vi "DAQ_Configure.vi"(6 "Dwell time (µs)":dbl, 7 "Scan XY (T) / i(t) (F)":bool, 8 "error in":errorcluster caption="entrée d'erreur", 9 "Position XY (for i(t))":dbl[](array[numeric]), 10 "Scanning positions":dbl[][](array[numeric]), 11 "Scanning cluster":T2={"Nx"=4, "Ny"=4, "# Repetition"=1, "FOV_X (µm)"=100.0, "FOV_Y (µm)"=100.0, "Calib_X"=0.1, "Calib_Y"=0.1, "Center X (µm)"=50.0, "Center_Y (µm)"=50.0, "Bi-directionnal?"=FALSE} {"# Repetition" min=1 step=1; "Ny" min=1 step=1; "Nx" min=1 step=1}) -> (0 "error out":errorcluster caption="sortie d'erreur", 3 "Task cluster":T1)   [LabVIEW 2026]
uses:
  <vilib>/DAQmx/write.llb/DAQmx Write (Analog 1D DBL NChan 1Samp).vi
  <vilib>/DAQmx/write.llb/DAQmx Write (Analog 2D DBL NChan NSamp).vi
  <vilib>/DAQmx/create/channels.llb/DAQmx Create Channel (CO-Pulse Generation-Frequency).vi
  <vilib>/DAQmx/configure/timing.llb/DAQmx Timing (Implicit).vi
  <vilib>/DAQmx/create/channels.llb/DAQmx Create Channel (AO-Voltage-Basic).vi
  <vilib>/DAQmx/miscellaneous.llb/DAQmx Fill In Error Info.vi
  <vilib>/DAQmx/configure/timing.llb/DAQmx Timing (Sample Clock).vi
  <vilib>/DAQmx/create/channels.llb/DAQmx Create Channel (AI-Voltage-Basic).vi
  <vilib>/DAQmx/configure/trigger.llb/DAQmx Start Trigger (Digital Edge).vi
  <vilib>/DAQmx/create/channels.llb/DAQmx Create Channel (CI-Pulse Width).vi
  <resource>/objmgr/daqmx.rc
panel:
  out "Pixel_Freq":dbl
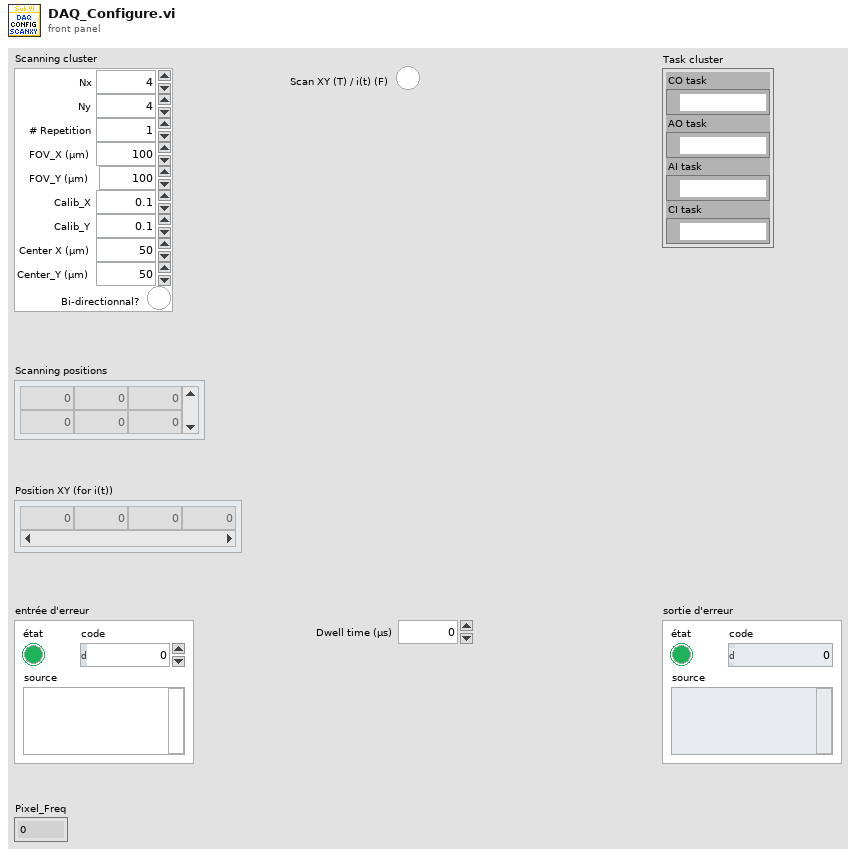
[diagram p1: front panel]
types:
  T1 = cluster{"CO task":refnum<k21>, "AO task":refnum<k21>, "AI task":refnum<k21>, "CI task":refnum<k21>}
  T2 = cluster{"Nx":u16, "Ny":u16, "# Repetition":u16, "FOV_X (µm)":dbl, "FOV_Y (µm)":dbl, "Calib_X":dbl, "Calib_Y":dbl, "Center X (µm)":dbl, "Center_Y (µm)":dbl, "Bi-directionnal?":bool}
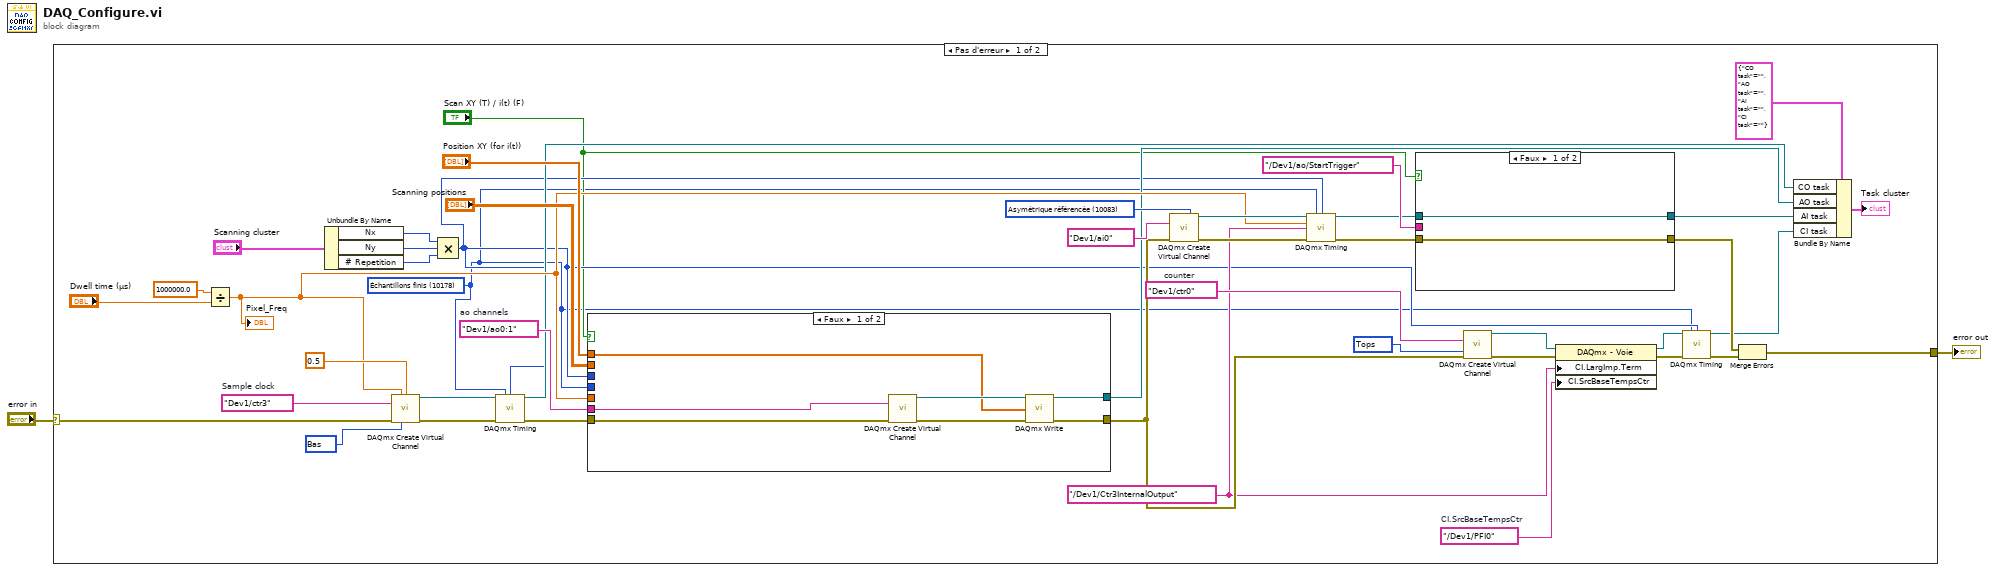
[diagram p0: block diagram]
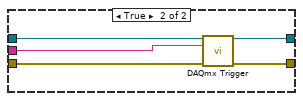
[diagram p2: hidden frame]
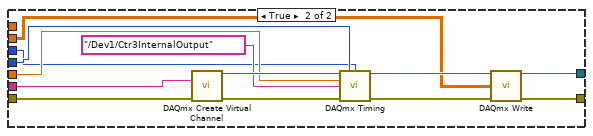
[diagram p3: hidden frame]
diagram:
  n1 = case shown="Pas d'erreur" "error in" {
    selector: "error in" -> [w45 w75]
    tunnel: [w19 w75] -> w1
    frame No Error {
      w15 = tag "/Dev1/PFI0"  # CI.SrcBaseTempsCtr
      w23 = 10304 items=["Secondes"=10364, "Tops"=10304, "D'une échelle personnalisée"=10065] ("units")
      w24 = tag "Dev1/ctr0"  # counter
      w18 = tag "/Dev1/Ctr3InternalOutput" ("source")
      w30 = 10083 items=["Par défaut"=-1, "Asymétrique référencée"=10083, "Asymétrique non référencée"=10078, "Différentielle"=10106, "Pseudodifférentielle"=12529] ("input terminal configuration")
      w37 = tag "Dev1/ao0:1"  # ao channels
      w3 = 10178 items=["Échantillons finis"=10178, "Échantillons continus"=10123, "Point par point avec cadencement matériel"=12522] ("sample mode")
      w40 = 10214 items=["Haut"=10192, "Bas"=10214] ("idle state")
      w42 = tag "Dev1/ctr3"  # Sample clock
      n2 = Divide(x=1000000.0, y="Dwell time (µs)") -> (x/y=w27:dbl)
      "Pixel_Freq" <- w27
      n3 = Unbundle By Name("Scanning cluster") -> ("Nx"=w34:u16, "Ny"=w33:u16, "# Repetition"=w32:u16)
      n4 = call-poly <vilib>:"DAQmx Create Virtual Channel.vi"("frequency"=w27, "duty cycle"=0.5 ("Duty cycle"), "counter"=w42, "error in"=w45, "idle state"=w40) -> ("task out"=w44:refnum<k21>, "error out"=w43:errorcluster)  [unwired: 9 in]
      n5 = Compound Arithmetic op=MULTIPLY(w34, w33, w32) -> (w5:u16)
      n6 = call-poly <vilib>:"DAQmx Timing.vi"("task/channels in"=w44, "sample mode"=w3, "samples per channel"=w5, "error in"=w43) -> ("task out"=w14:refnum<k21>, "error out"=w39:errorcluster)  [unwired: 10 in]
      n7 = case shown="Faux" "Scan XY (T) / i(t) (F)" {
        tunnel: w39 -> [w60 w74]
        tunnel: w27 -> [_ w70]
        tunnel: w3 -> [_ w69]
        tunnel: w5 -> [_ w68]
        tunnel: [w56 w65] -> w25
        tunnel: "Scanning positions" -> [_ w64]
        tunnel: w37 -> [w61 w63]
        tunnel: "Position XY (for i(t))" -> [w57 _]
        tunnel: [w55 w62] -> w11
        frame False {
          n8 = call-poly <vilib>:"DAQmx Create Virtual Channel.vi"("physical channels"=w61, "error in"=w60) -> ("task out"=w59:refnum<k21>, "error out"=w58:errorcluster)  [unwired: 12 in]
          n9 = call-poly <vilib>:"DAQmx Write.vi"("task/channels in"=w59, "data"=w57, "error in"=w58) -> ("task out"=w55:refnum<k21>, "error out"=w56:errorcluster)  [unwired: 10 in, 1 out]
        }
        frame True {
          n10 = call-poly <vilib>:"DAQmx Create Virtual Channel.vi"("physical channels"=w63, "error in"=w74) -> ("task out"=w72:refnum<k21>, "error out"=w73:errorcluster)  [unwired: 12 in]
          n11 = call-poly <vilib>:"DAQmx Timing.vi"("task/channels in"=w72, "sample mode"=w69, "samples per channel"=w68, "rate"=w70, "source"=tag "/Dev1/Ctr3InternalOutput", "error in"=w73) -> ("task out"=w67:refnum<k21>, "error out"=w66:errorcluster)  [unwired: 8 in]
          n12 = call-poly <vilib>:"DAQmx Write.vi"("task/channels in"=w67, "data"=w64, "error in"=w66) -> ("task out"=w62:refnum<k21>, "error out"=w65:errorcluster)  [unwired: 10 in, 1 out]
        }
      }
      n13 = call-poly <vilib>:"DAQmx Create Virtual Channel.vi"("input terminal configuration"=w30, "physical channels"=tag "Dev1/ai0", "error in"=w25) -> ("task out"=w29:refnum<k21>, "error out"=w28:errorcluster)  [unwired: 11 in]
      n14 = call-poly <vilib>:"DAQmx Timing.vi"("task/channels in"=w29, "sample mode"=w3, "samples per channel"=w5, "rate"=w27, "source"=w18, "error in"=w28) -> ("task out"=w9:refnum<k21>, "error out"=w8:errorcluster)  [unwired: 8 in]
      n15 = case shown="Faux" "Scan XY (T) / i(t) (F)" {
        tunnel: tag "/Dev1/ao/StartTrigger" ("source") -> [_ w54]
        tunnel: [w48 w53] -> w20
        tunnel: [w49 w52] -> w10
        tunnel: w9 -> [w49 w51]
        tunnel: w8 -> [w48 w50]
        frame False {
        }
        frame True {
          n16 = call-poly <vilib>:"DAQmx Trigger.vi"("task/channels in"=w51, "source"=w54, "error in"=w50) -> ("task out"=w52:refnum<k21>, "error out"=w53:errorcluster)  [unwired: 11 in]
        }
      }
      n17 = call-poly <vilib>:"DAQmx Create Virtual Channel.vi"("counter"=w24, "units"=w23, "error in"=w25) -> ("task out"=w21:refnum<k21>, "error out"=w22:errorcluster)  [unwired: 11 in]
      n18 = property class="DAQmx - Voie"(reference=w21, error in=w22, "CI.LargImp.Term"=w18, "CI.SrcBaseTempsCtr"=w15) -> (reference out=w17:refnum<k21>, error out=w16:errorcluster)
      n19 = call-poly <vilib>:"DAQmx Timing.vi"("task/channels in"=w17, "sample mode"=w3, "samples per channel"=w5, "error in"=w16) -> ("task out"=w7:refnum<k21>, "error out"=w6:errorcluster)  [unwired: 10 in]
      n20 = Merge Errors(w20, w6) -> (w19:errorcluster)
      n21 = Bundle By Name(cluster=T1 {"CO task"="", "AO task"="", "AI task"="", "CI task"=""} ("cluster d'entrée"), "CO task"=w14, "AO task"=w11, "AI task"=w10, "CI task"=w7) -> (→"Task cluster":T1)
    }
    frame Error {
    }
  }
  "error out" <- w1
